vi "BASE.Device.GetState.vi"(8 "error in (no error)":errorcluster, 11 "BASE.Device in":refnum<class "BASE.Device.lvclass">) -> (0 "error out":errorcluster, 2 "config":T1, 3 "BASE.Device out":refnum<class "BASE.Device.lvclass">)   [LabVIEW 2019]
uses:
  BASE.Device.lvclass
  C:/Repos/KLA-Demo/Source/Subsystems/BASE/BASE/BASE.lvclass
  D:/Program Files (x86)/National Instruments/LabVIEW 2019/vi.lib/ActorFramework/Actor/Actor.lvclass
  config--cluster.ctl
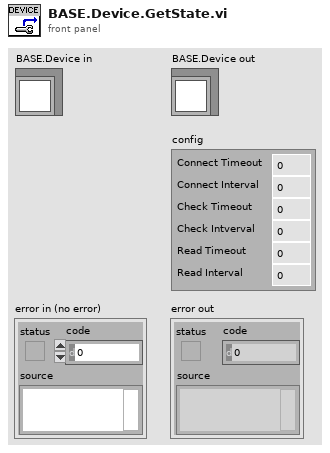
[diagram p1: front panel]
types:
  T1 = typedef "BASE.Device.lvlib/BASE.Device.lvclass/config--cluster.ctl" = cluster{"Connect Timeout":i32, "Connect Interval":u32, "Check Timeout":i32, "Check Intverval":u32, "Read Timeout":i32, "Read Interval":u32}
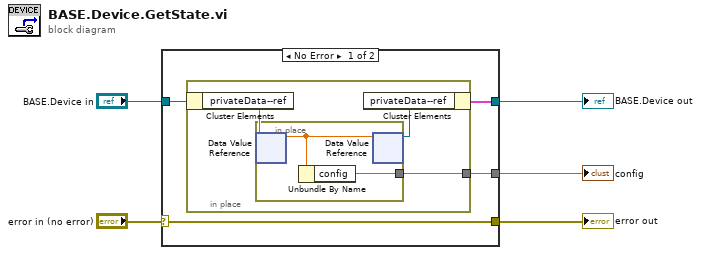
[diagram p0: block diagram]
diagram:
  n1 = case shown="No Error" "error in (no error)" {
    selector: "error in (no error)" -> [w9 w15]
    tunnel: [w9 w15] -> w1
    tunnel: [w6 w16] -> w3
    tunnel: "BASE.Device in" -> [w7 w16]
    tunnel: [w8 _] -> w2
    frame No Error {
      n2 = in-place {
        in-place-border: [w12] -> w8
        n3 = in-place-cluster #1(w7) -> ("privateData--ref"=w11)
        n4 = in-place {
          in-place-border: [w14] -> w12
          n5 = in-place-dvr #2(w11) -> (w13:dbl)  [unwired: 1 out]
          n6 = Unbundle By Name(w13) -> ("config"=w14)
          n7 = in-place-dvr #2(w13) -> (w10:refnum<data-value>)  [unwired: 1 out]
        }
        n8 = in-place-cluster #1("privateData--ref"=w10) -> (w6:cluster{})
      }
    }
    frame Error {
    }
  }
  "error out" <- w1
  "BASE.Device out" <- w3
  "config" <- w2
